vi "DSF.Shared.Configuration.Framework.Cluster to Objects.vi"(8 "error in (no error)":errorcluster, 11 "Framework Configuration in":refnum<class "DSF.Shared.Configuration.Framework.lvclass">) -> (0 "error out":errorcluster, 3 "Framework Configuration out":refnum<class "DSF.Shared.Configuration.Framework.lvclass">)   [LabVIEW 2017, in "DSF.Engine.lvlib" / "DSF.Shared.Configuration.Framework.lvclass"]
uses:
  DSF.Shared.Configuration.Framework.lvclass
  DSF.Shared.Configuration.Framework.lvclass/DSF.Shared.Configuration.Framework.ctl
  Plugin/DSF.Shared.Configuration.Plugin.lvclass
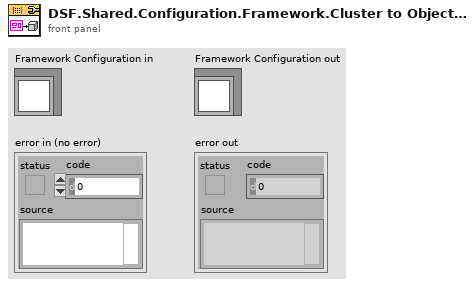
[diagram p1: front panel]
types:
  T1 = typedef "DSF Configuration API.lvlib/DSF Engine Framework Configuration.ctl" = cluster{"Plugins":T2[]}
  T2 = typedef "DSF Configuration API.lvlib/DSF Engine Plugin Configuration.ctl" = cluster{"name":string, "class":string, "cycle timing":T3, "Transfer Groups":T4[], "settings":T10}
  T3 = typedef "DSF Configuration API.lvlib/DSF Timing Info.ctl" = cluster{"priority":i32, "decimation":i32, "offset":i32}
  T4 = typedef "DSF Configuration API.lvlib/DSF Engine Transfer Group Configuration.ctl" = cluster{"name":string, "direction":T5, "cycle timing":T3, "Transfers":T6[], "settings":T10}
  T5 = typedef "DSF Configuration API.lvlib/DSF Direction.ctl" = enum8{"Tx", "Rx"}
  T6 = typedef "DSF Configuration API.lvlib/DSF Engine Transfer Configuration.ctl" = cluster{"name":string, "byte order":T7, "channel configurations":T8[], "settings":T10}
  T7 = typedef "DSF Configuration API.lvlib/DSF Byte Order.ctl" = enum8{"big-endian", "little-endian"}
  T8 = typedef "DSF Configuration API.lvlib/DSF Engine Channel Configuration.ctl" = cluster{"name":string, "data type":T9, "count":u64, "buffer offset":u64, "engine offset":u64, "settings":T10}
  T9 = typedef "DSF Configuration API.lvlib/DSF Data Type.ctl" = enum8{"Bool", "SGL", "DBL", "I8", "I16", "I32", "I64", "U8", "U16", "U32", "U64"}
  T10 = typedef "DSF Configuration API.lvlib/DSF Settings Info.ctl" = cluster{"key":string, "value":string}[]
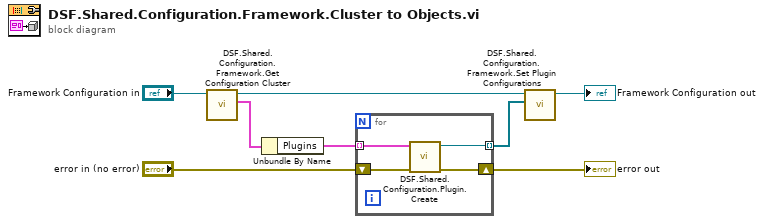
[diagram p0: block diagram]
diagram:
  n1 = call "DSF.Shared.Configuration.Framework.Get Configuration Cluster.vi"("Framework Configuration in"="Framework Configuration in") -> ("Framework Configuration"=w7:T1, "Framework Configuration out"=w3:refnum<class "DSF.Shared.Configuration.Framework.lvclass">)  [unwired: 9 in]
  n2 = Unbundle By Name(w7) -> ("Plugins"=w6:T2[])
  n3 = for {
    tunnel: w6 -> [w12] mode=indexing
    tunnel: [w11] -> w1 mode=indexing
    shift-right: [w10] -> w5
    shift-left: "error in (no error)" -> [w9]
    n4 = call "DSF.Shared.Configuration.Plugin.Create.vi"("error in (no error)"=w9, "Plugin Configuration cluster"=w12) -> ("error out"=w10:errorcluster, "Plugin Configuration"=w11:refnum<class "DSF.Shared.Configuration.Plugin.lvclass">)  [unwired: 8 in]
  }
  "error out" <- w5
  n5 = call "DSF.Shared.Configuration.Framework.Set Plugin Configurations.vi"("Plugin Configurations"=w1, "Framework Configuration in"=w3) -> ("Framework Configuration out"=→"Framework Configuration out":refnum<class "DSF.Shared.Configuration.Framework.lvclass">)  [unwired: 9 in]
